vi "dispose.vi"(8 "error in (no error)":errorcluster, 11 "IBaseObject in":refnum<class "IBaseObject.lvclass">) -> (0 "error out":errorcluster, 3 "IBaseObject out":refnum<class "IBaseObject.lvclass">)   [LabVIEW 2022 SP3, in "openDAQ.lvlib" / "IBaseObject.lvlib" / "IBaseObject.lvclass"]
uses:
  <instrlib>/openDAQ/Public/Classes/IBaseObject/IBaseObject.lvclass
  <instrlib>/openDAQ/Public/Classes/IBaseObject/IBaseObject.lvclass/IBaseObject.ctl
  <instrlib>/openDAQ/Binaries/Windows/x86/copendaq32.dll
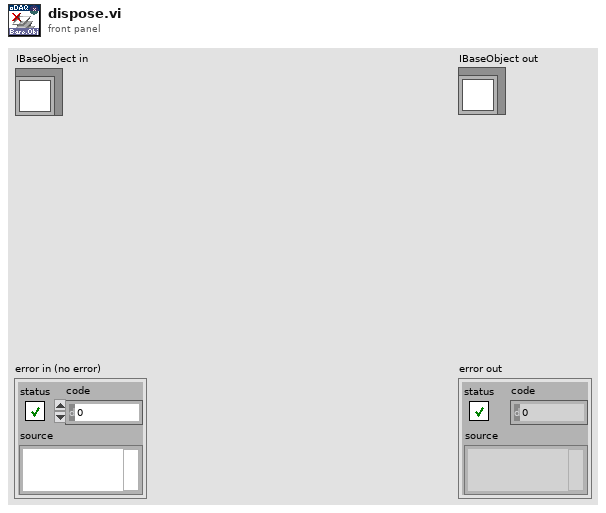
[diagram p1: front panel]
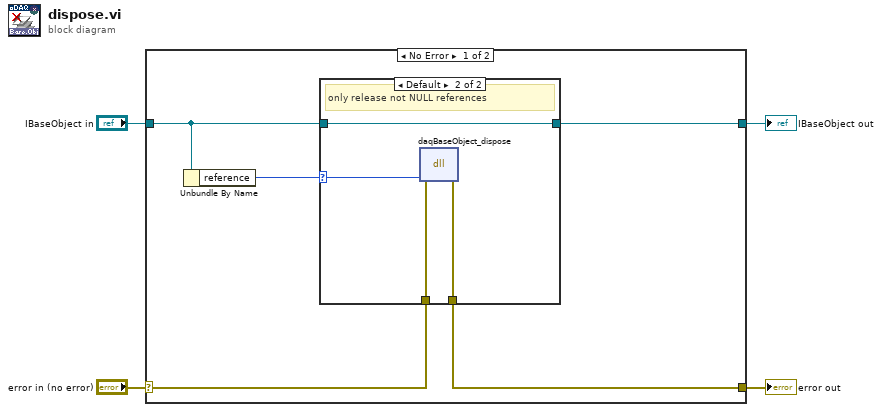
[diagram p0: block diagram]
diagram:
  n1 = case shown="No Error" "error in (no error)" {
    selector: "error in (no error)" -> [w9 w17]
    tunnel: [w8 w17] -> w3
    tunnel: "IBaseObject in" -> [w6 w16]
    tunnel: [w5 w16] -> w1
    frame No Error {
      n2 = Unbundle By Name(w6) -> ("reference"=w7:i64)
      n3 = case shown="Default" w7 {
        selector: w7 -> [_ w13]
        tunnel: w9 -> [w11 w15]
        tunnel: [w11 w14] -> w8
        tunnel: w6 -> [w10 w12]
        tunnel: [w10 w12] -> w5
        frame 0 {
        }
        frame Default {
          # "only release not NULL references"
          n4 = dll-call lib="C:/Program Files (x86)/National Instruments/LabVIEW 2022/instr.lib/openDAQ/Binaries/Windows/x86/copendaq*.*" fn="daqBaseObject_dispose"(error in=w15, "reference"=w13) -> (error out=w14:errorcluster)  [unwired: 4 in, 1 out]
        }
      }
    }
    frame Error {
    }
  }
  "error out" <- w3
  "IBaseObject out" <- w1
